vi "SetSingleShot.vi"(8 "error in":errorcluster, 11 "VISA resource":refnum<visa-resource-name>) -> (0 "error out":errorcluster)   [LabVIEW 2011]
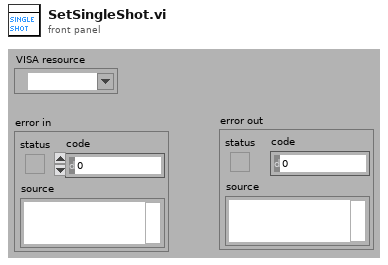
[diagram p1: front panel]
types:
  T1 = enum16{"Initialize", "Write", "Write/Read", "Read", "Clear", "Close"}
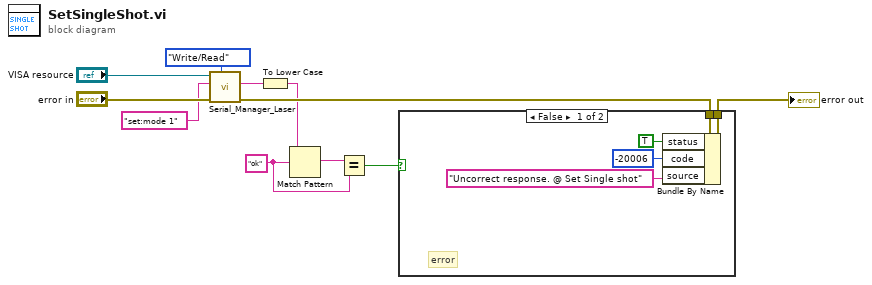
[diagram p0: block diagram]
diagram:
  w3 = "ok" ("read buffer")
  n1 = call "Serial_Manager_Laser.vi"("Job"=T1."Write/Read", "error in"="error in", "write buffer"="set:mode 1", "VISA resource"="VISA resource") -> ("error out"=w7:errorcluster, "read buffer"=w6:string)  [unwired: 6 in]
  n2 = To Lower Case(string=w6) -> (all lower case string=w5:string)
  n3 = Match Pattern(string=w5, regular expression=w3) -> (match substring=w4:string)  [unwired: 1 in, 3 out]
  n4 = Equal?(x=w4, y=w3) -> (x = y?=w2:bool)
  n5 = case shown="False" w2 {
    tunnel: w7 -> [w16 w17]
    tunnel: [w15 w17] -> w11
    frame False {
      # "error"
      n6 = Bundle By Name(cluster=w16, "status"=TRUE, "code"=-20006, "source"="Uncorrect response. @ Set Single shot") -> (w15:errorcluster)
    }
    frame True {
    }
  }
  "error out" <- w11
